vi "Sample_NotificationBufferedRead.vi"() -> ()   [LabVIEW 2022 SP3, in "ADS_Library.lvlib"]
doc: "ADS Read single symbol notifications\n\n- The Example illustrates a sample block diagram for 1 ADS symbols.\n- The ADS Symbol is registered in a separate thread.\n- A reader waits for notifications in a separate thread. As soon the notifications are received, they are written directly inside client-side LVBuffer. The reader waits for a certain timeout in milliseconds (infinite if -1) to move the samples inside LVBuffer to LabVIEW™. The size of samples is defined by LVBufferSize during symbol configuration.\n- The Notifications can be stopped after an <b>ElapseTime in milliseconds</b> or can run infinite time."
uses:
  <userlib>/Beckhoff-LabVIEW-Interface/Utilities/Notification/Buffered User-Event Data.ctl
  <userlib>/Beckhoff-LabVIEW-Interface/_DependsOn/Base/Read/Register LVB-Notification.vi
  ADS_Library.lvlib
panel:
  in  "XMLDescription":string
  out "SymbolName":string
  out "Buffer Data":T1 {"RawData" format="%x"; "Timestamps" format="%x"}
  out "DataBytes":u32
  out "ElementsInQueue":u32
  out "bTimeout":bool
  # "%"
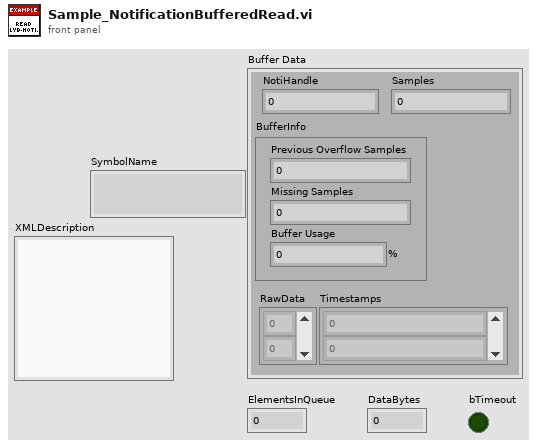
[diagram p1: front panel]
types:
  T1 = typedef "Buffered User-Event Data.ctl" = cluster{"NotiHandle":u32, "Samples":i32, "BufferInfo":cluster{"Previous Overflow Samples":u32, "Missing Samples":u32, "Buffer Usage":dbl}, "RawData":u8[], "Timestamps":i64[]}
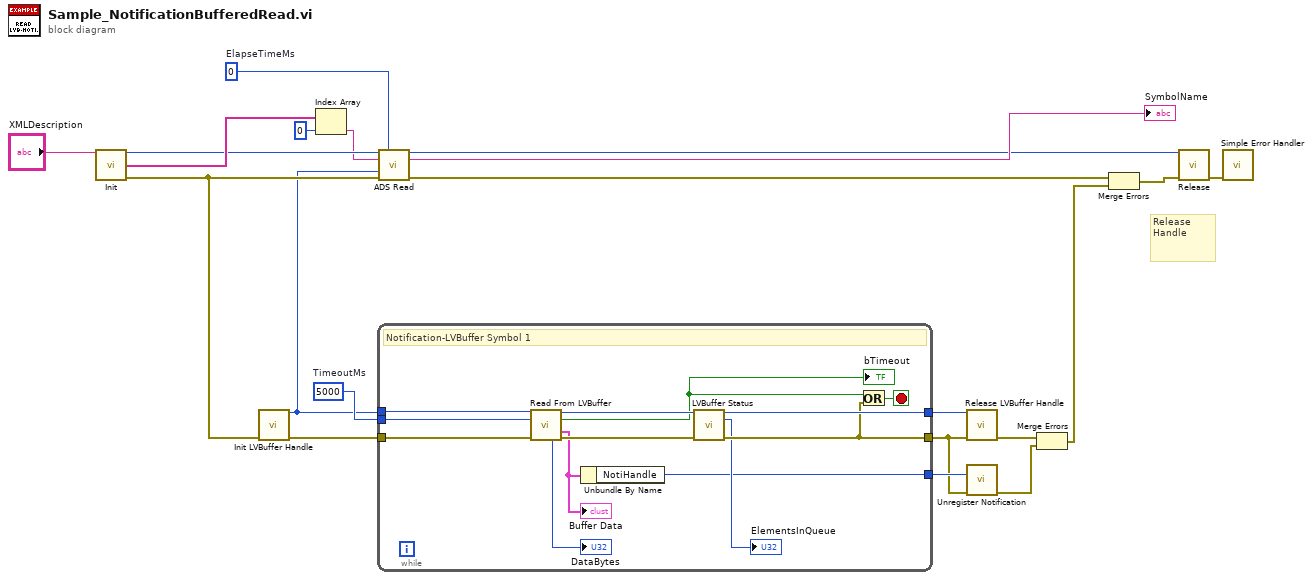
[diagram p0: block diagram]
diagram:
  w9 = 0  # ElapseTimeMs
  w17 = 5000  # TimeoutMs
  # "Release\nHandle"
  n1 = call <userlib>:"Init.vi"("XMLDescription"="XMLDescription") -> ("Handle"=w10:u32, "ReadGrpSymbols"=w11:string[], "error out"=w12:errorcluster)  [unwired: 10 in, 2 out]
  n2 = call <userlib>:"Init LVBuffer Handle.vi"("error constant"=w12) -> ("Buffer Handle"=w6:u32, "error IO"=w21:errorcluster)  [unwired: 13 in]
  n3 = Index Array(array=w11, index=0) -> (element=w7:string)
  n4 = while {
    tunnel: w21 -> [w34]
    tunnel: [w28] -> w15
    tunnel: w6 -> [w32]
    tunnel: [w30] -> w18
    tunnel: w17 -> [w29]
    tunnel: [w22] -> w16
    stop <- w33 stop-if-true
    # "Notification-LVBuffer Symbol 1"
    n5 = call <userlib>:"Read From LVBuffer.vi"("Buffer Handle"=w32, "TimeoutMs"=w29, "error constant"=w34) -> ("Buffer Handle"=w31:u32, "bTimeout"=w26:bool, "Buffer Data"=w23:T1, "DataBytes"=→"DataBytes":u32, "error IO"=w25:errorcluster)  [unwired: 8 in]
    "bTimeout" <- w26
    "Buffer Data" <- w23
    n6 = Unbundle By Name(w23) -> ("NotiHandle"=w22:u32)
    n7 = call <userlib>:"LVBuffer Status.vi"("Buffer Handle"=w31, "error constant"=w25) -> ("Buffer Handle"=w30:u32, "Elements In Buffer"=→"ElementsInQueue":u32, "error IO"=w28:errorcluster)  [unwired: 11 in]
    n8 = Or(x=w26, y=w28) -> (x .or. y?=w33:bool)
  }
  n9 = call-poly <userlib>:"ADS Read.vi"("Handle"=w10, "ElapseTimeMs"=w9, "SymbolName"=w7, "LVBuffer Handle"=w6, "error in (no error)"=w12) -> ("Handle"=w1:u32, "SymbolName"=→"SymbolName":string, "error out"=w20:errorcluster)  [unwired: 8 in]
  n10 = call <userlib>:"Release LVBuffer Handle.vi"("Buffer Handle"=w18, "error constant"=w15) -> ("error IO"=w19:errorcluster)  [unwired: 13 in]
  n11 = call <userlib>:"Unregister Notification.vi"("Reader Handle"=w16, "error in"=w15) -> ("error out"=w13:errorcluster)  [unwired: 10 in, 3 out]
  n12 = Merge Errors(w19, w13) -> (w14:errorcluster)
  n13 = Merge Errors(w20, w14) -> (w2:errorcluster)
  n14 = call <userlib>:"Release.vi"("Handle"=w1, "error in (no error)"=w2) -> ("error out"=w3:errorcluster)  [unwired: 13 in]
  n15 = call <vilib>:"Simple Error Handler.vi"("error in (no error)"=w3) -> ()  [unwired: 4 in, 5 out]
